vi "p1.vi"() -> ()   [LabVIEW 2025, in "d5.lvlib"]
uses:
  d5.lvlib
  AOC/AOC.lvlib
panel:
  out "Answer":i64
  in  "Example":string="3-5\n10-14\n16-20\n12-18\n\n1\n5\n8\n11\n17\n32"
  in  "Example":bool
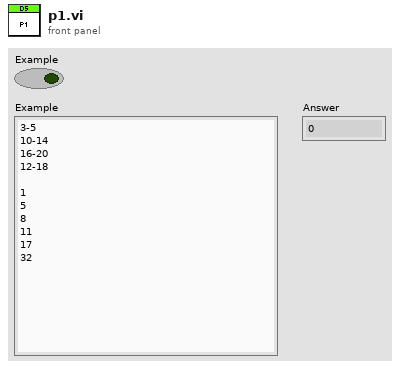
[diagram p1: front panel]
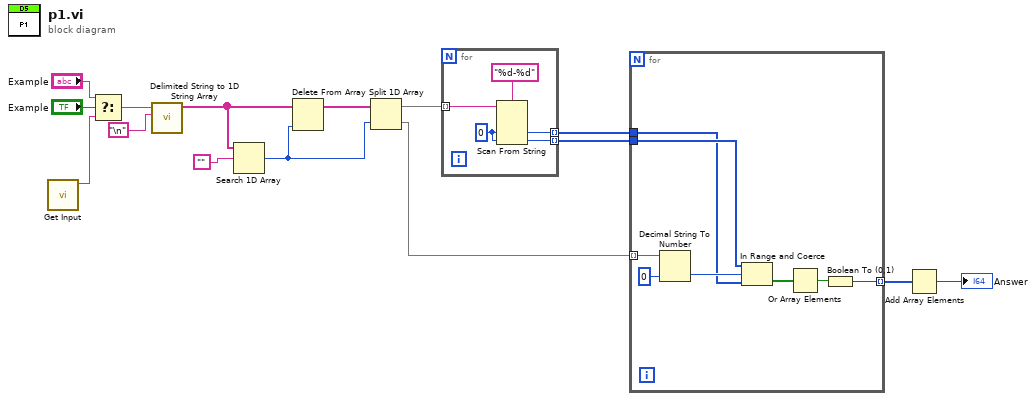
[diagram p0: block diagram]
diagram:
  n1 = call "Get Input.vi"() -> ("Input"=w13:string)  [unwired: 11 in]
  n2 = Select(t="Example", s="Example", f=w13) -> (s? t:f=w12:string)
  n3 = call <vilib>:"Delimited String to 1D String Array.vi"("delimiter"="\n", "delimited string"=w12) -> ("string array"=w8:string[])  [unwired: 9 in]
  n4 = Search 1D Array(1D array=w8, element="") -> (index of element=w6:i32)  [unwired: 1 in]
  n5 = Delete From Array(array=w8, index=w6) -> (array with subset deleted=w7:string[])  [unwired: 1 in, 1 out]
  n6 = Split 1D Array(array=w7, index=w6) -> (first subarray=w5:string[], second subarray=w4:string[])
  n7 = for {
    tunnel: w5 -> [w20] mode=indexing
    tunnel: [w17] -> w2 mode=indexing
    tunnel: [w16] -> w3 mode=indexing
    w18 = i64 0 ("default value 14")
    n8 = Scan From String(format string="%d-%d", input string=w20, default 1=w18, default 2=w18) -> (output 1=w17:i64, output 2=w16:i64)  [unwired: 2 in, 3 out]
  }
  n9 = for {
    tunnel: w4 -> [w28] mode=indexing
    tunnel: w3 -> [w26]
    tunnel: w2 -> [w25]
    tunnel: [w22] -> w1 mode=indexing
    n10 = Decimal String To Number(string=w28, default (0L)=i64 0 ("default (0 I32)")) -> (number=w27:i64)  [unwired: 1 in, 1 out]
    n11 = In Range and Coerce(upper limit=w26, x=w27, lower limit=w25) -> (In Range?=w24:bool[])  [unwired: 1 out]
    n12 = Or Array Elements(Boolean array=w24) -> (logical OR=w23:bool)
    n13 = Boolean To (0,1)(Boolean=w23) -> (0, 1=w22:i16)
  }
  n14 = Add Array Elements(numeric array=w1) -> (sum=→"Answer":i16)
